vi "dataCommon.vi"(8 "error in (no error)":errorcluster, 11 "Command Text":string) -> (0 "error out":errorcluster, 3 "Data":string[][](array[string]))   [LabVIEW 2014]
uses:
  <vilib>/addons/database/NI_Database_API.lvlib
  <vilib>/addons/database/Connection.llb/DB Tools Open Connec (String).vi
  <vilib>/addons/database/Connection.llb/Conn Execute.vi
  <vilib>/addons/database/Recordset.llb/Rec Destroy - Connection.vi
panel:
  in  "error in (no error) 2":errorcluster
  out "error out 2":errorcluster
  in  "SQL query":string
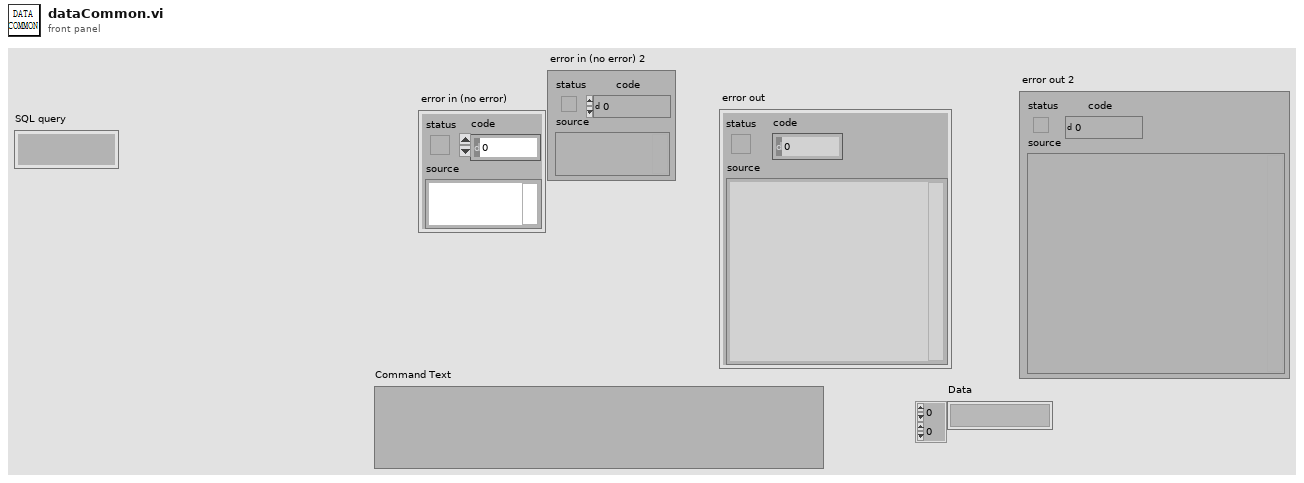
[diagram p1: front panel]
types:
  T1 = enum32{"invalid app kind", "Development System", "Run Time System", "Student Edition", "Embedded LabVIEW", "Evaluation", "Custom"}
  T2 = typedef "NI_Database_API.lvlib/Conn ObjectReference.ctl" = refnum<k1>
  T3 = typedef "NI_Database_API.lvlib/Rec ObjectReference.ctl" = refnum<k1>
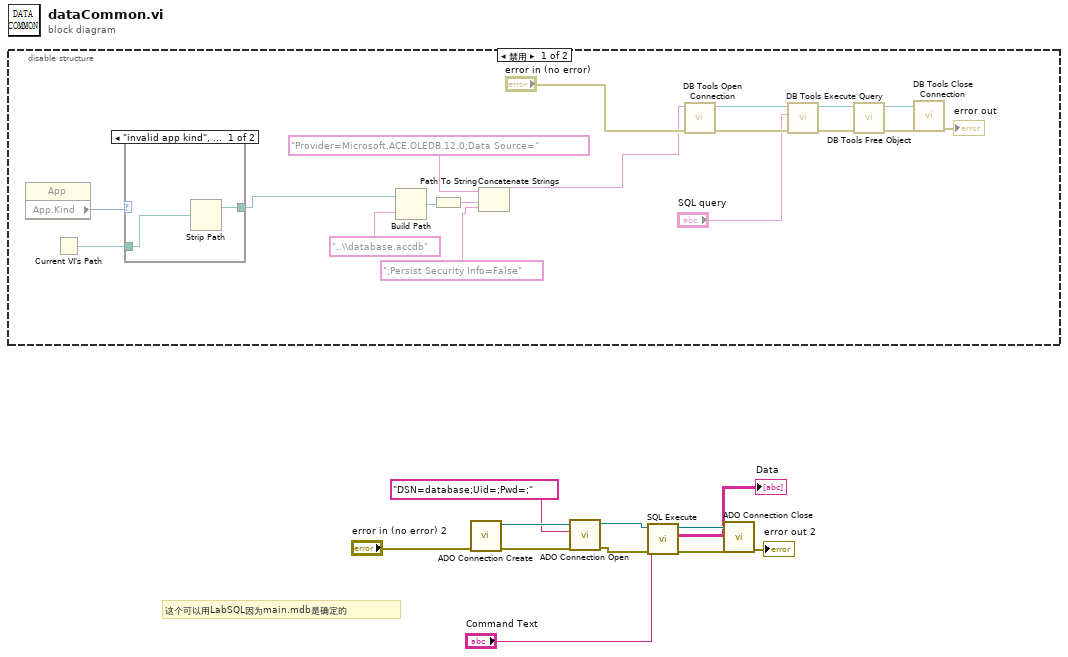
[diagram p0: block diagram]
diagram:
  # "这个可以用LabSQL因为main.mdb是确定的"
  n1 = disable-structure shown="禁用" {
    frame Disabled {
      n2 = property class="App"() -> ("App.Kind"=w13:T1)  [unwired: 2 in, 2 out]
      n3 = Current VI's Path() -> (path=w14:path)
      n4 = case shown="\"invalid app kind\", 默认" w13 {
        tunnel: w14 -> [w31 w32]
        tunnel: [w30 w32] -> w15
        frame "invalid app kind", Default {
          n5 = Strip Path(path=w31) -> (stripped path=w30:path)  [unwired: 1 out]
        }
        frame "Development System" {
        }
      }
      n6 = Build Path(base path=w15, name or relative path="..\\database.accdb" ("名称或相对路径")) -> (appended path=w17:path)
      n7 = Path To String(path=w17) -> (string=w18:string)
      n8 = Concatenate Strings("Provider=Microsoft.ACE.OLEDB.12.0;Data Source=", w18, ";Persist Security Info=False") -> (w27:string)
      n9 = call-poly <vilib>:"DB Tools Open Connection.vi"("error in (no error)"="error in (no error)", "connection information"=w27) -> ("error out"=w25:errorcluster, "connection reference"=w26:T2)  [unwired: 6 in]
      n10 = call-poly <vilib>:"DB Tools Execute Query.vi"("error in (no error)"=w25, "SQL query"="SQL query", "connection reference"=w26) -> ("error out"=w23:errorcluster, "recordset reference"=w24:T3)  [unwired: 5 in]
      n11 = call-poly <vilib>:"DB Tools Free Object.vi"("error in (no error)"=w23, "recordset reference"=w24) -> ("error out"=w21:errorcluster, "connection reference"=w22:T2)  [unwired: 8 in]
      n12 = call <vilib>:"DB Tools Close Connection.vi"("error in (no error)"=w21, "connection reference"=w22) -> ("error out"=→"error out":errorcluster)  [unwired: 5 in]
    }
    frame Enabled {
    }
  }
  n13 = call <userlib>:"ADO Connection Create.vi"("error in (no error)"="error in (no error) 2") -> ("error out"=w10:errorcluster, "ADODB._Connection Out"=w11:refnum<k7>)  [unwired: 9 in]
  n14 = call <userlib>:"ADO Connection Open.vi"("error in (no error)"=w10, "ConnectionString"="DSN=database;Uid=;Pwd=;", "ADODB._Connection In"=w11) -> ("error out"=w7:errorcluster, "ADODB._Connection Out"=w8:refnum<k7>)  [unwired: 7 in]
  n15 = call <userlib>:"SQL Execute.vi"("error in (no error)"=w7, "Command Text"="Command Text", "ADODB._Connection In"=w8) -> ("error out"=w5:errorcluster, "Data"=→"Data":string[][], "ADODB._Connection Out"=w6:refnum<k7>)  [unwired: 5 in, 1 out]
  n16 = call <userlib>:"ADO Connection Close.vi"("error in (no error)"=w5, "ADODB._Connection In"=w6) -> ("error out"=→"error out 2":errorcluster)  [unwired: 8 in, 1 out]
